vi "CMAP_Example.vi"() -> ()   [LabVIEW 2018]
uses:
  <vilib>/Utility/file.llb/Read Delimited Spreadsheet (DBL).vi
panel:
  in  "STOP":bool
  in  "start":dbl(slide) scale=0.0..255.0
  in  "end":dbl(slide)=1.0 scale=0.0..255.0
  out "Intensity Graph":dbl[][](graph)
  in  "file path (dialog if empty)":path
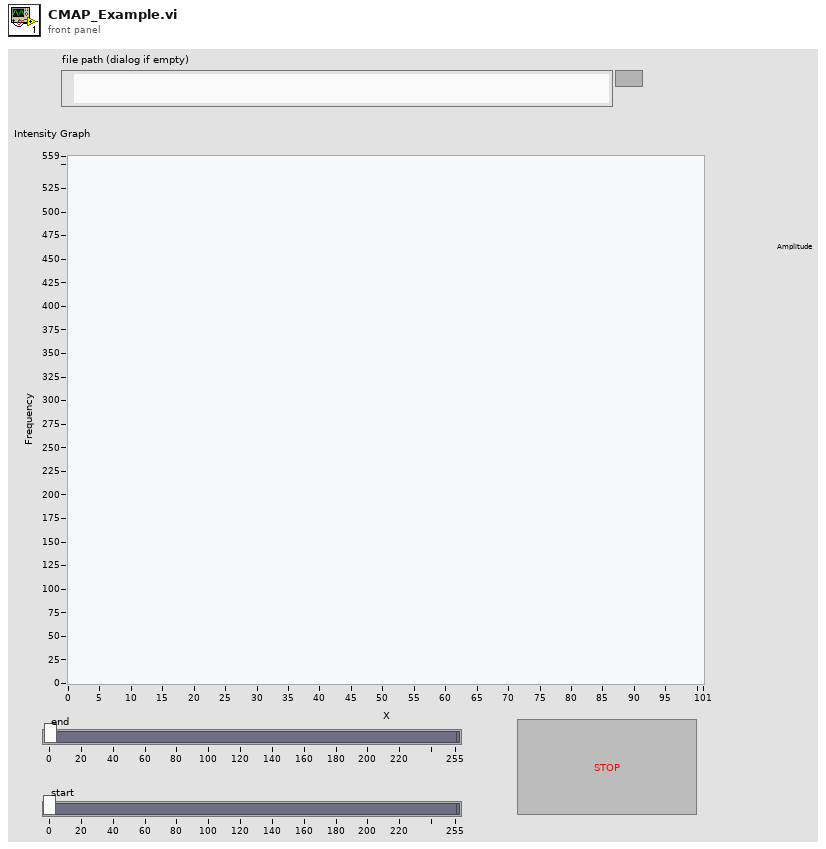
[diagram p1: front panel]
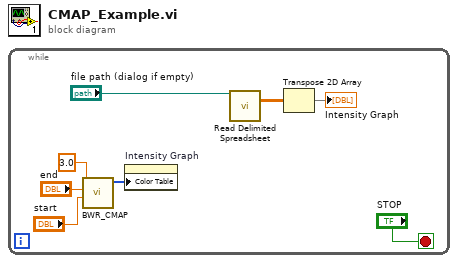
[diagram p0: block diagram]
diagram:
  n1 = while {
    stop <- "STOP" stop-if-true
    n2 = call "BWR_CMAP.vi"("Brightness"="start", "Contrast"="end", "Delta"=3.0) -> ("Cmap array"=w5:u32[])  [unwired: 8 in]
    n3 = property on="Intensity Graph" class="IntGraph (strict)"("Color Table"=w5) -> ()  [unwired: 2 in, 2 out]
    n4 = call-poly <vilib>:"Read Delimited Spreadsheet.vi"("file path (dialog if empty)"="file path (dialog if empty)") -> ("all rows"=w7:dbl[][])  [unwired: 9 in, 5 out]
    n5 = Transpose 2D Array(2D array=w7) -> (transposed array=→"Intensity Graph":dbl[][])
  }
